vi "TESTik.vi"() -> ()   [LabVIEW 2018]
uses:
  3_amp_volt.lvclass
panel:
  in  "stop":bool
  out "Waveform Chart 2":sgl[][](graph)
  out "Waveform Chart":sgl[][](graph)
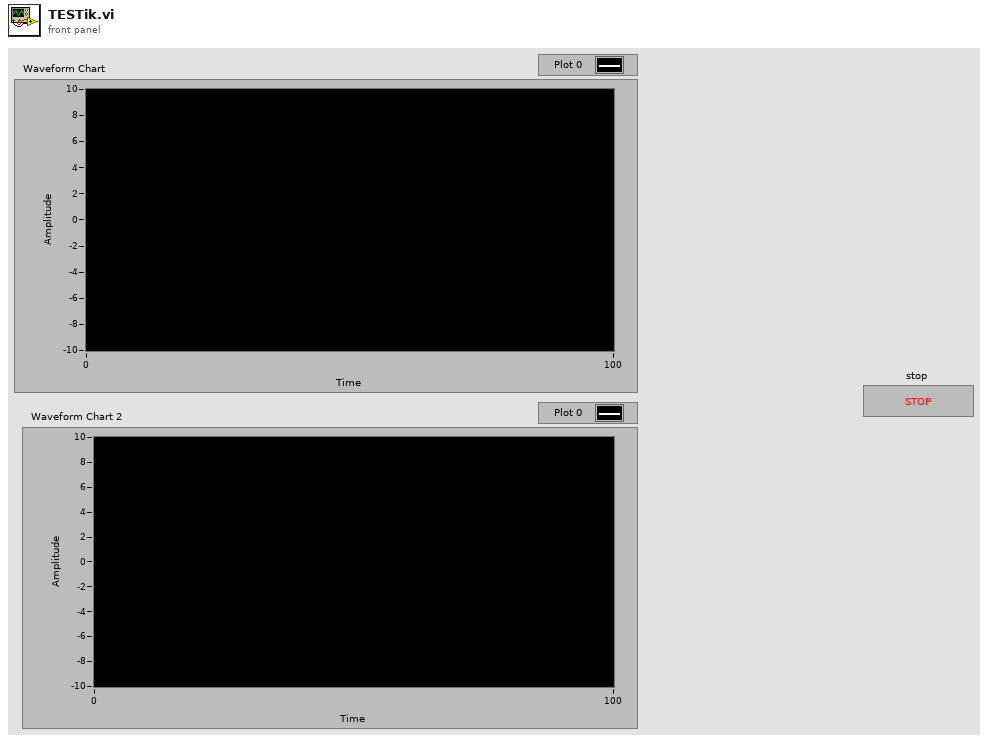
[diagram p1: front panel]
types:
  T1 = cluster{"VISA resource name":refnum<visa-resource-name>, u8}[]
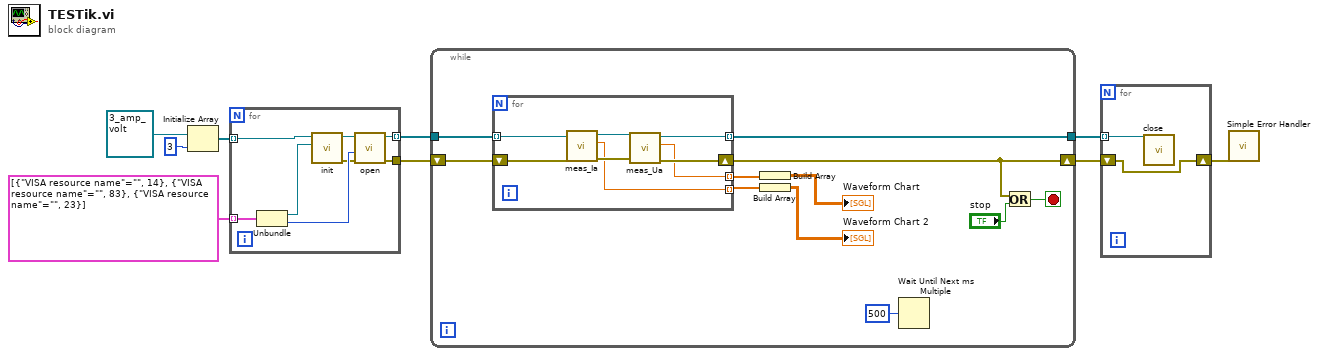
[diagram p0: block diagram]
diagram:
  n1 = Initialize Array(refnum<class "3_amp_volt.lvclass"> refnum ("3_amp_volt.lvclass"), 3 ("dimension size")) -> (w6:refnum<class "3_amp_volt.lvclass">[])
  n2 = for {
    tunnel: T1 [{"VISA resource name"="", 14}, {"VISA resource name"="", 83}, {"VISA resource name"="", 23}] -> [w17] mode=indexing
    tunnel: w6 -> [w16] mode=indexing
    tunnel: [w11] -> w5 mode=indexing
    tunnel: [w10] -> w4
    n3 = Unbundle(w17) -> ("VISA resource name"=w15:refnum<visa-resource-name>, w13:u8)
    n4 = call "init.vi"("VISA resource name"=w15, "3_amp_volt in"=w16) -> ("error out"=w12:errorcluster, "3_amp_volt out"=w14:refnum<class "3_amp_volt.lvclass">)  [unwired: 8 in]
    n5 = call "open.vi"("3_amp_volt in"=w14, "Slave ID"=w13, "error in (no error)"=w12) -> ("3_amp_volt out"=w11:refnum<class "3_amp_volt.lvclass">, "error out"=w10:errorcluster)  [unwired: 6 in]
  }
  n6 = while {
    tunnel: w5 -> [w28]
    shift-right: [w21] -> w2
    shift-left: w4 -> [w27]
    tunnel: [w26] -> w3
    stop <- w19 stop-if-true
    n7 = for {
      tunnel: w28 -> [w33] mode=indexing
      shift-right: [w35] -> w21
      shift-left: w27 -> [w31]
      tunnel: [w36] -> w26 mode=indexing
      tunnel: [w34] -> w25 mode=indexing
      tunnel: [w29] -> w24 mode=indexing
      n8 = call "meas_Ia.vi"("error in (no error)"=w31, "3_amp_volt in"=w33) -> ("error out"=w30:errorcluster, "Measured Ia"=w29:sgl, "3_amp_volt out"=w32:refnum<class "3_amp_volt.lvclass">)  [unwired: 7 in]
      n9 = call "meas_Ua.vi"("error in (no error)"=w30, "3_amp_volt in"=w32) -> ("error out"=w35:errorcluster, "Measured Ua"=w34:sgl, "3_amp_volt out"=w36:refnum<class "3_amp_volt.lvclass">)  [unwired: 7 in]
    }
    n10 = Build Array(w25) -> (→"Waveform Chart":sgl[][])
    n11 = Build Array(w24) -> (→"Waveform Chart 2":sgl[][])
    n12 = Wait Until Next ms Multiple(millisecond multiple=u32 500) -> ()  [unwired: 1 out]
    n13 = Or(x=w21, y="stop") -> (x .or. y?=w19:bool)
  }
  n14 = for {
    tunnel: w3 -> [w38] mode=indexing
    shift-right: [w37] -> w1
    shift-left: w2 -> [w37]
    n15 = call "close.vi"("3_amp_volt in"=w38) -> ()  [unwired: 9 in, 2 out]
  }
  n16 = call <vilib>:"Simple Error Handler.vi"("error in (no error)"=w1) -> ()  [unwired: 4 in, 5 out]
